vi "FdxCmdTxUDPBlockWriteCvi.vi"(8 "error in":errorcluster, 9 "UdpBlockWriteMsgArray":u32[](array[numeric]), 10 "MsgCount":u32, 11 "InstrumentHandle":u32) -> (0 "error out":errorcluster, 1 "UdpBlockWriteResultArray":u32[](array[numeric]), 2 "GlobalResultCode":i32, 3 "InstrumentHandle":u32, 4 "MsgCountOut":u32)   [LabVIEW 2020, in "AIM664LV.lvlib"]
doc: "This function is used to write a pure message to one or more UDP ports. The ports can be a sampling or a queuing port AFDX Communication port. If the data size is not applicable for the data size associated to this port, this function will return an error.\nFor sampling ports this function initializes / modifies data contents.\nFor queuing ports a transmission is initiated when data is written to a UDP port if the tranmitter is running.\nThis function can be used if the transmitter is running or not running.\nFor sampling ports this function should be called before the port is started to initialize the data contents of the sampling port."
uses:
  AIM664LV.lvlib
  AFDX_LibraryAdmin/FdxGlobalDllPath.vi
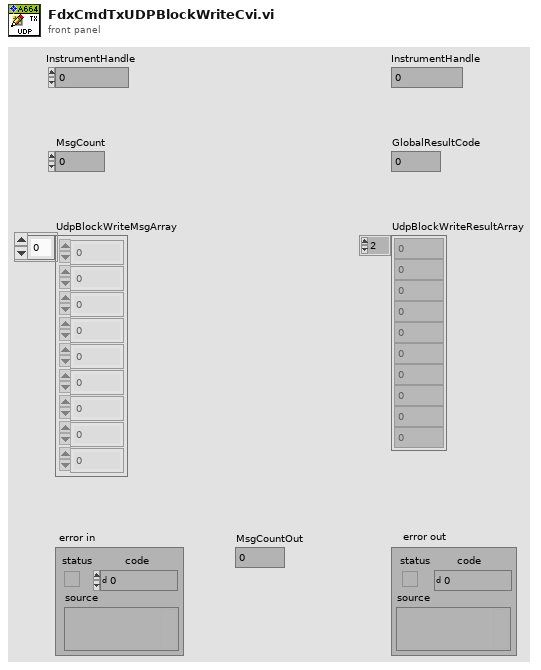
[diagram p1: front panel]
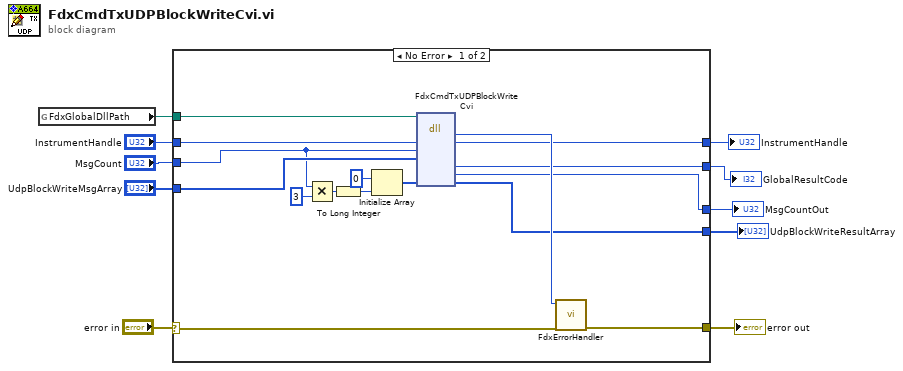
[diagram p0: block diagram]
diagram:
  n1 = global read "FdxGlobalDllPath.vi" "FdxGlobalDllPath"() -> (w8:path)
  n2 = case shown="No Error" "error in" {
    selector: "error in" -> [w25 w28]
    tunnel: [w26 w28] -> w10
    tunnel: w8 -> [w18 _]
    tunnel: [w17 w27] -> w7
    tunnel: "InstrumentHandle" -> [w16 w27]
    tunnel: [w15 _] -> w5
    tunnel: [w14 _] -> w4
    tunnel: "UdpBlockWriteMsgArray" -> [w13 _]
    tunnel: [w12 _] -> w2
    tunnel: "MsgCount" -> [w11 _]
    frame No Error {
      n3 = Multiply(x=w11, y=u32 3) -> (x*y=w20:u32)
      n4 = To Long Integer(number=w20) -> (32bit integer=w19:i32)
      n5 = Initialize Array(u32 0 ("element"), w19) -> (w23:u32[])
      n6 = dll-call lib="aim_fdx.19.dll" fn="FdxCmdTxUDPBlockWriteCvi"(path in=w18, "InstrumentHandle"=w16, "MsgCount"=w11, "UdpBlockWriteMsgArray"=w13, "UdpBlockWriteResultArray"=w23) -> ("status"=w24:i32, "InstrumentHandle"=w17:u32, "GlobalResultCode"=w15:i32, "MsgCountOut"=w14:u32, "UdpBlockWriteResultArray"=w12:u32[])  [unwired: 6 in, 2 out]
      n7 = call "FdxErrorHandler.vi"("error in"=w25, "AIM Error"=w24) -> ("error out"=w26:errorcluster)  [unwired: 9 in]
    }
    frame Error {
    }
  }
  "error out" <- w10
  "InstrumentHandle" <- w7
  "UdpBlockWriteResultArray" <- w2
  "GlobalResultCode" <- w5
  "MsgCountOut" <- w4
